vi "Field vs Slow IV v2.vi"() -> ()   [LabVIEW 2023]
uses:
  <vilib>/Utility/file.llb/Write Delimited Spreadsheet (DBL).vi
panel:
  in  "Tab Control 2":enum32{"cRIO", "Lockin", "Plot 2", "Plot 3"}(tab)
  out "I vs AI":cluster{"Y":dbl[], "Y":dbl[]}[](graph)=[{"Y"=[0.0, 0.01, 0.02, 0.03, 0.04, 0.05, 0.06, 0.07, 0.08, 0.09, 0.1, 0.11, 0.12, 0.13, 0.14, 0.15, 0.16, 0.17, 0.18, 0.19, 0.2, 0.21, 0.22, 0.23, 0.24, 0.25, 0.26, 0.27, 0.28, 0.29, 0.3, 0.31, 0.32, 0.33, 0.34, 0.35000000000000003, 0.36, 0.37, 0.38, 0.39, 0.4, 0.41000000000000003, 0.42, 0.43, 0.44, 0.45, 0.46, 0.47000000000000003, 0.48, 0.49, 0.5, 0.51, 0.52, 0.53, 0.54, 0.55, 0.56, 0.5700000000000001, 0.58, 0.59, 0.6, 0.61, 0.62, 0.63, 0.64, 0.65, 0.66, 0.67, 0.68, 0.6900000000000001, 0.7000000000000001, 0.71, 0.72, 0.73, 0.74, 0.75, 0.76, 0.77, 0.78, 0.79, 0.8, 0.81, 0.8200000000000001, 0.8300000000000001, 0.84, 0.85, 0.86, 0.87, 0.88, 0.89, 0.9, 0.91, 0.92, 0.93, 0.9400000000000001, 0.9500000000000001, 0.96, 0.97, 0.98, 0.99, 1.0, 1.01, 1.02, 1.03, 1.04, 1.05, 1.06, 1.07, 1.08, 1.09, 1.1, 1.11, 1.12, 1.1300000000000001, 1.1400000000000001, 1.1500000000000001, 1.16, 1.17, 1.18, 1.19, 1.2, 1.21, 1.22, 1.23, 1.24, 1.25, 1.26, 1.27, 1.28, 1.29, 1.3, 1.31, 1.32, 1.33, 1.34, 1.35, 1.36, 1.37, 1.3800000000000001, 1.3900000000000001, 1.4000000000000001, 1.41, 1.42, 1.43, 1.44, 1.45, 1.46, 1.47, 1.48, 1.49, 1.5, 1.51, 1.52, 1.53, 1.54, 1.55, 1.56, 1.57, 1.58, 1.59, 1.6, 1.61, 1.62, 1.6300000000000001, 1.6400000000000001, 1.6500000000000001, 1.6600000000000001, 1.67, 1.68, 1.69, 1.7, 1.71, 1.72, 1.73, 1.74, 1.75, 1.76, 1.77, 1.78, 1.79, 1.8, 1.81, 1.82, 1.83, 1.84, 1.85, 1.86, 1.87, 1.8800000000000001, 1.8900000000000001, 1.9000000000000001, 1.9100000000000001, 1.92, 1.93, 1.94, 1.95, 1.96, 1.97, 1.98, 1.99, 2.0, 2.0100000000000002, 2.02, 2.0300000000000002, 2.04, 2.05, 2.06, 2.07, 2.08, 2.09, 2.1, 2.11, 2.12, 2.13, 2.14, 2.15, 2.16, 2.17, 2.18, 2.19, 2.2, 2.21, 2.22, 2.23, 2.24, 2.25, 2.2600000000000002, 2.27, 2.2800000000000002, 2.29, 2.3000000000000003, 2.31, 2.32, 2.33, 2.34, 2.35, 2.36, 2.37, 2.38, 2.39, 2.4, 2.41, 2.42, 2.43, 2.44, 2.45, 2.46, 2.47, 2.48, 2.49, 2.5, 2.5100000000000002, 2.52, 2.5300000000000002, 2.54, 2.5500000000000003, 2.56, 2.57, 2.58, 2.59, 2.6, 2.61, 2.62, 2.63, 2.64, 2.65, 2.66, 2.67, 2.68, 2.69, 2.7, 2.71, 2.72, 2.73, 2.74, 2.75, 2.7600000000000002, 2.77, 2.7800000000000002, 2.79, 2.8000000000000003, 2.81, 2.82, 2.83, 2.84, 2.85, 2.86, 2.87, 2.88, 2.89, 2.9, 2.91, 2.92, 2.93, 2.94, 2.95, 2.96, 2.97, 2.98, 2.99, 3.0], "Y"=[2.09912109375e-05, 2.6015625e-05, 2.0756835937500003e-05, 2.4968261718750003e-05, 2.291015625e-05, 2.5644531250000002e-05, 2.3308105468750003e-05, 2.341796875e-05, 2.62646484375e-05, 2.48876953125e-05, 2.1000976562500003e-05, 2.4147949218750003e-05, 2.5754394531250003e-05, 2.3442382812500002e-05, 2.462890625e-05, 2.25537109375e-05, 2.5007324218750002e-05, 2.3037109375000003e-05, 2.2856445312500002e-05, 2.2717285156250002e-05, 2.41357421875e-05, 2.44873046875e-05, 2.4709472656250002e-05, 2.421630859375e-05, 2.6560058593750003e-05, 2.137451171875e-05, 2.361083984375e-05, 2.473876953125e-05, 1.990478515625e-05, 2.388427734375e-05, 2.21875e-05, 2.4270019531250003e-05, 2.480712890625e-05, 2.262451171875e-05, 2.370849609375e-05, 2.3144531250000002e-05, 2.422607421875e-05, 2.44775390625e-05, 2.233642578125e-05, 2.346923828125e-05, 2.3159179687500003e-05, 2.3681640625e-05, 2.5126953125000003e-05, 2.4238281250000002e-05, 2.0891113281250002e-05, 2.25927734375e-05, 2.1511230468750002e-05, 2.44482421875e-05, 2.1755371093750002e-05, 2.4130859375e-05, 2.342041015625e-05, 2.7426757812500002e-05, 2.2099609375e-05, 2.27001953125e-05, 2.5681152343750005e-05, 2.5070800781250004e-05, 2.67138671875e-05, 1.97119140625e-05, 2.027587890625e-05, 2.1047363281250002e-05, 2.325439453125e-05, 2.8649902343750002e-05, 2.2717285156250002e-05, 2.348876953125e-05, 2.63134765625e-05, 2.3552246093750003e-05, 2.6933593750000004e-05, 2.6767578125000004e-05, 2.558837890625e-05, 2.342041015625e-05, 2.642822265625e-05, 2.598388671875e-05, 2.4238281250000002e-05, 3.224609375e-05, 2.9941406250000003e-05, 3.089111328125e-05, 2.904541015625e-05, 4.072998046875e-05, 3.9006347656250006e-05, 4.6594238281250005e-05, 5.4602050781250004e-05, 5.186767578125e-05, 5.7617187500000004e-05, 5.64990234375e-05, 5.828125e-05, 6.0437011718750005e-05, 6.245361328125e-05, 6.554443359375e-05, 6.246826171875e-05, 6.654052734375e-05, 6.34423828125e-05, 6.683349609375e-05, 6.337158203124999e-05, 6.903076171875e-05, 7.051513671875001e-05, 6.797119140625e-05, 7.292724609375001e-05, 7.169433593750001e-05, 7.08251953125e-05, 7.458740234375e-05, 7.213134765625e-05, 7.000732421875e-05, 7.192626953125e-05, 7.560791015625e-05, 7.204833984375e-05, 7.61279296875e-05, 7.792236328125e-05, 7.745849609375e-05, 7.70068359375e-05, 7.795410156250001e-05, 8.091796875e-05, 8.347412109375e-05, 8.00830078125e-05, 7.839111328125001e-05, 8.351562500000001e-05, 8.119384765625e-05, 7.959716796875001e-05, 7.7822265625e-05, 8.2099609375e-05, 8.49853515625e-05, 8.425537109375001e-05, 8.463867187500001e-05, 8.37744140625e-05, 8.5576171875e-05, 8.346435546875e-05, 8.697509765625e-05, 8.865234375e-05, 8.927978515625e-05, 8.916748046875001e-05, 8.64404296875e-05, 9.275634765625001e-05, 9.026611328125001e-05, 9.218017578125e-05, 8.979003906250001e-05, 9.381103515625001e-05, 9.07177734375e-05, 9.376953125000001e-05, 9.364990234375001e-05, 9.407470703125001e-05, 9.20556640625e-05, 9.776611328125001e-05, 9.44970703125e-05, 9.7314453125e-05, 9.900390625e-05, 9.63671875e-05, 0.00010056884765625, 9.861572265625e-05, 0.00010073974609375001, 0.0001025146484375, 0.00010167480468750001, 0.0001015673828125, 0.00010302490234375, 0.00010155517578125, 0.00010652587890625001, 0.00010431152343750002, 0.0001023779296875, 0.0001060400390625, 0.00010368164062500001, 0.00010692382812500002, 0.0001058544921875, 0.0001072802734375, 0.00010769287109375001, 0.00010914306640625, 0.00010889892578125, 0.00010593505859375002, 0.00011151123046875001, 0.000111650390625, 0.00010907958984374999, 0.00011219482421875, 0.00010731201171875, 0.00011229248046875, 0.00011305664062500001, 0.0001139501953125, 0.00011421142578125001, 0.0001163134765625, 0.00011355224609375002, 0.000115390625, 0.0001179736328125, 0.000118828125, 0.00011745361328124999, 0.00012102294921875001, 0.00011634033203125002, 0.00011909912109375001, 0.00012057861328125, 0.00011787841796875001, 0.00012433349609375, 0.00012124267578125001, 0.00012028076171875, 0.00011879882812500001, 0.00012194335937500001, 0.0001228076171875, 0.00012369873046875, 0.00012751708984375, 0.00012575927734375002, 0.00012471923828125, 0.000126513671875, 0.0001298388671875, 0.00013156982421875003, 0.00013070068359375, 0.0001272998046875, 0.00013069091796875002, 0.00012986083984375003, 0.00013344970703125, 0.000129853515625, 0.00013442138671875, 0.00013176269531250002, 0.00013392822265625, 0.0001347265625, 0.0001333251953125, 0.00013612060546875, 0.0001330517578125, 0.00013523681640625, 0.00013681152343750002, 0.000135244140625, 0.00013745849609375, 0.00013937988281250002, 0.00013837646484375, 0.00014040771484375, 0.00014029785156250001, 0.00014124755859375, 0.00013885986328125, 0.00013990478515625001, 0.00013862060546875, 0.000142509765625, 0.00014126220703125002, 0.00014351318359375002, 0.00014447265625000002, 0.000145751953125, 0.00014315185546875, 0.00014501220703125, 0.00014614990234375, 0.0001438818359375, 0.00014447265625000002, 0.0001490283203125, 0.00014803466796875001, 0.0001479296875, 0.00014945800781250001, 0.0001504296875, 0.0001508837890625, 0.00015038085937500002, 0.00015168212890625, 0.00015281982421875, 0.00015464599609375, 0.0001536572265625, 0.00015431884765625, 0.00015674804687499999, 0.0001547314453125, 0.00015652587890625002, 0.00015684326171875001, 0.00015552734374999999, 0.00015493408203125003, 0.00015597900390625, 0.000159130859375, 0.00015770751953125, 0.00016166015625000002, 0.00016299560546875001, 0.00016100341796875, 0.00015983642578125, 0.00016435546875, 0.000161025390625, 0.0001635986328125, 0.0001652197265625, 0.00016124755859375, 0.00016710205078125, 0.00016457275390625, 0.00016589111328125, 0.000166328125, 0.0001637353515625, 0.00016878662109375, 0.00016859619140625, 0.0001676611328125, 0.00016881835937500002, 0.00016962646484375, 0.0001681005859375, 0.00017082031250000002, 0.00017445556640625, 0.0001698876953125, 0.0001721630859375, 0.00017332275390625001, 0.00017365966796875003, 0.0001742822265625, 0.000175556640625, 0.00017460937500000001, 0.00017539306640625003, 0.00017764404296875, 0.000178935546875, 0.00017882324218750003, 0.00018162353515625002, 0.00017995117187500002, 0.00017988037109375, 0.00017955566406250003, 0.00017959228515625002, 0.000180078125, 0.00018293212890625, 0.00017876953125, 0.00018194091796875001, 0.0001847021484375, 0.00018335205078125002, 0.000184111328125, 0.00018517822265625, 0.0001835205078125]}, ...(4 in all)]
  out "Name 0":string="DC Voltage V"
  out "I vs R":cluster{"Y":dbl[], "Y":dbl[]}[](graph)=[{"Y"=[0.0, 0.01, 0.02, 0.03, 0.04, 0.05, 0.06, 0.07, 0.08, 0.09, 0.1, 0.11, 0.12, 0.13, 0.14, 0.15, 0.16, 0.17, 0.18, 0.19, 0.2, 0.21, 0.22, 0.23, 0.24, 0.25, 0.26, 0.27, 0.28, 0.29, 0.3, 0.31, 0.32, 0.33, 0.34, 0.35000000000000003, 0.36, 0.37, 0.38, 0.39, 0.4, 0.41000000000000003, 0.42, 0.43, 0.44, 0.45, 0.46, 0.47000000000000003, 0.48, 0.49, 0.5, 0.51, 0.52, 0.53, 0.54, 0.55, 0.56, 0.5700000000000001, 0.58, 0.59, 0.6, 0.61, 0.62, 0.63, 0.64, 0.65, 0.66, 0.67, 0.68, 0.6900000000000001, 0.7000000000000001, 0.71, 0.72, 0.73, 0.74, 0.75, 0.76, 0.77, 0.78, 0.79, 0.8, 0.81, 0.8200000000000001, 0.8300000000000001, 0.84, 0.85, 0.86, 0.87, 0.88, 0.89, 0.9, 0.91, 0.92, 0.93, 0.9400000000000001, 0.9500000000000001, 0.96, 0.97, 0.98, 0.99, 1.0, 1.01, 1.02, 1.03, 1.04, 1.05, 1.06, 1.07, 1.08, 1.09, 1.1, 1.11, 1.12, 1.1300000000000001, 1.1400000000000001, 1.1500000000000001, 1.16, 1.17, 1.18, 1.19, 1.2, 1.21, 1.22, 1.23, 1.24, 1.25, 1.26, 1.27, 1.28, 1.29, 1.3, 1.31, 1.32, 1.33, 1.34, 1.35, 1.36, 1.37, 1.3800000000000001, 1.3900000000000001, 1.4000000000000001, 1.41, 1.42, 1.43, 1.44, 1.45, 1.46, 1.47, 1.48, 1.49, 1.5, 1.51, 1.52, 1.53, 1.54, 1.55, 1.56, 1.57, 1.58, 1.59, 1.6, 1.61, 1.62, 1.6300000000000001, 1.6400000000000001, 1.6500000000000001, 1.6600000000000001, 1.67, 1.68, 1.69, 1.7, 1.71, 1.72, 1.73, 1.74, 1.75, 1.76, 1.77, 1.78, 1.79, 1.8, 1.81, 1.82, 1.83, 1.84, 1.85, 1.86, 1.87, 1.8800000000000001, 1.8900000000000001, 1.9000000000000001, 1.9100000000000001, 1.92, 1.93, 1.94, 1.95, 1.96, 1.97, 1.98, 1.99, 2.0, 2.0100000000000002, 2.02, 2.0300000000000002, 2.04, 2.05, 2.06, 2.07, 2.08, 2.09, 2.1, 2.11, 2.12, 2.13, 2.14, 2.15, 2.16, 2.17, 2.18, 2.19, 2.2, 2.21, 2.22, 2.23, 2.24, 2.25, 2.2600000000000002, 2.27, 2.2800000000000002, 2.29, 2.3000000000000003, 2.31, 2.32, 2.33, 2.34, 2.35, 2.36, 2.37, 2.38, 2.39, 2.4, 2.41, 2.42, 2.43, 2.44, 2.45, 2.46, 2.47, 2.48, 2.49, 2.5, 2.5100000000000002, 2.52, 2.5300000000000002, 2.54, 2.5500000000000003, 2.56, 2.57, 2.58, 2.59, 2.6, 2.61, 2.62, 2.63, 2.64, 2.65, 2.66, 2.67, 2.68, 2.69, 2.7, 2.71, 2.72, 2.73, 2.74, 2.75, 2.7600000000000002, 2.77, 2.7800000000000002, 2.79, 2.8000000000000003, 2.81, 2.82, 2.83, 2.84, 2.85, 2.86, 2.87, 2.88, 2.89, 2.9, 2.91, 2.92, 2.93, 2.94, 2.95, 2.96, 2.97, 2.98, 2.99, 3.0], "Y"=[0.0, 0.0, 0.0, 0.0, 0.0, 0.0, 0.0, 0.0, 0.0, 0.0, 0.0, 0.0, 0.0, 0.0, 0.0, 0.0, 0.0, 0.0, 0.0, 0.0, 0.0, 0.0, 0.0, 0.0, 0.0, 0.0, 0.0, 0.0, 0.0, 0.0, 0.0, 0.0, 0.0, 0.0, 0.0, 0.0, 0.0, 0.0, 0.0, 0.0, 0.0, 0.0, 0.0, 0.0, 0.0, 0.0, 0.0, 0.0, 0.0, 0.0, 0.0, 0.0, 0.0, 0.0, 0.0, 0.0, 0.0, 0.0, 0.0, 0.0, 0.0, 0.0, 0.0, 0.0, 0.0, 0.0, 0.0, 0.0, 0.0, 0.0, 0.0, 0.0, 0.0, 0.0, 0.0, 0.0, 0.0, 0.0, 0.0, 0.0, 0.0, 0.0, 0.0, 0.0, 0.0, 0.0, 0.0, 0.0, 0.0, 0.0, 0.0, 0.0, 0.0, 0.0, 0.0, 0.0, 0.0, 0.0, 0.0, 0.0, 0.0, 0.0, 0.0, 0.0, 0.0, 0.0, 0.0, 0.0, 0.0, 0.0, 0.0, 0.0, 0.0, 0.0, 0.0, 0.0, 0.0, 0.0, 0.0, 0.0, 0.0, 0.0, 0.0, 0.0, 0.0, 0.0, 0.0, 0.0, 0.0, 0.0, 0.0, 0.0, 0.0, 0.0, 0.0, 0.0, 0.0, 0.0, 0.0, 0.0, 0.0, 0.0, 0.0, 0.0, 0.0, 0.0, 0.0, 0.0, 0.0, 0.0, 0.0, 0.0, 0.0, 0.0, 0.0, 0.0, 0.0, 0.0, 0.0, 0.0, 0.0, 0.0, 0.0, 0.0, 0.0, 0.0, 0.0, 0.0, 0.0, 0.0, 0.0, 0.0, 0.0, 0.0, 0.0, 0.0, 0.0, 0.0, 0.0, 0.0, 0.0, 0.0, 0.0, 0.0, 0.0, 0.0, 0.0, 0.0, 0.0, 0.0, 0.0, 0.0, 0.0, 0.0, 0.0, 0.0, 0.0, 0.0, 0.0, 0.0, 0.0, 0.0, 0.0, 0.0, 0.0, 0.0, 0.0, 0.0, 0.0, 0.0, 0.0, 0.0, 0.0, 0.0, 0.0, 0.0, 0.0, 0.0, 0.0, 0.0, 0.0, 0.0, 0.0, 0.0, 0.0, 0.0, 0.0, 0.0, 0.0, 0.0, 0.0, 0.0, 0.0, 0.0, 0.0, 0.0, 0.0, 0.0, 0.0, 0.0, 0.0, 0.0, 0.0, 0.0, 0.0, 0.0, 0.0, 0.0, 0.0, 0.0, 0.0, 0.0, 0.0, 0.0, 0.0, 0.0, 0.0, 0.0, 0.0, 0.0, 0.0, 0.0, 0.0, 0.0, 0.0, 0.0, 0.0, 0.0, 0.0, 0.0, 0.0, 0.0, 0.0, 0.0, 0.0, 0.0, 0.0, 0.0, 0.0, 0.0, 0.0, 0.0, 0.0, 0.0, 0.0, 0.0, 0.0, 0.0, 0.0, 0.0, 0.0, 0.0, 0.0, 0.0, 0.0, 0.0, 0.0, 0.0, 0.0, 0.0, 0.0]}, {"Y"=[0.0, 0.01, 0.02, 0.03, 0.04, 0.05, 0.06, 0.07, 0.08, 0.09, 0.1, 0.11, 0.12, 0.13, 0.14, 0.15, 0.16, 0.17, 0.18, 0.19, 0.2, 0.21, 0.22, 0.23, 0.24, 0.25, 0.26, 0.27, 0.28, 0.29, 0.3, 0.31, 0.32, 0.33, 0.34, 0.35000000000000003, 0.36, 0.37, 0.38, 0.39, 0.4, 0.41000000000000003, 0.42, 0.43, 0.44, 0.45, 0.46, 0.47000000000000003, 0.48, 0.49, 0.5, 0.51, 0.52, 0.53, 0.54, 0.55, 0.56, 0.5700000000000001, 0.58, 0.59, 0.6, 0.61, 0.62, 0.63, 0.64, 0.65, 0.66, 0.67, 0.68, 0.6900000000000001, 0.7000000000000001, 0.71, 0.72, 0.73, 0.74, 0.75, 0.76, 0.77, 0.78, 0.79, 0.8, 0.81, 0.8200000000000001, 0.8300000000000001, 0.84, 0.85, 0.86, 0.87, 0.88, 0.89, 0.9, 0.91, 0.92, 0.93, 0.9400000000000001, 0.9500000000000001, 0.96, 0.97, 0.98, 0.99, 1.0, 1.01, 1.02, 1.03, 1.04, 1.05, 1.06, 1.07, 1.08, 1.09, 1.1, 1.11, 1.12, 1.1300000000000001, 1.1400000000000001, 1.1500000000000001, 1.16, 1.17, 1.18, 1.19, 1.2, 1.21, 1.22, 1.23, 1.24, 1.25, 1.26, 1.27, 1.28, 1.29, 1.3, 1.31, 1.32, 1.33, 1.34, 1.35, 1.36, 1.37, 1.3800000000000001, 1.3900000000000001, 1.4000000000000001, 1.41, 1.42, 1.43, 1.44, 1.45, 1.46, 1.47, 1.48, 1.49, 1.5, 1.51, 1.52, 1.53, 1.54, 1.55, 1.56, 1.57, 1.58, 1.59, 1.6, 1.61, 1.62, 1.6300000000000001, 1.6400000000000001, 1.6500000000000001, 1.6600000000000001, 1.67, 1.68, 1.69, 1.7, 1.71, 1.72, 1.73, 1.74, 1.75, 1.76, 1.77, 1.78, 1.79, 1.8, 1.81, 1.82, 1.83, 1.84, 1.85, 1.86, 1.87, 1.8800000000000001, 1.8900000000000001, 1.9000000000000001, 1.9100000000000001, 1.92, 1.93, 1.94, 1.95, 1.96, 1.97, 1.98, 1.99, 2.0, 2.0100000000000002, 2.02, 2.0300000000000002, 2.04, 2.05, 2.06, 2.07, 2.08, 2.09, 2.1, 2.11, 2.12, 2.13, 2.14, 2.15, 2.16, 2.17, 2.18, 2.19, 2.2, 2.21, 2.22, 2.23, 2.24, 2.25, 2.2600000000000002, 2.27, 2.2800000000000002, 2.29, 2.3000000000000003, 2.31, 2.32, 2.33, 2.34, 2.35, 2.36, 2.37, 2.38, 2.39, 2.4, 2.41, 2.42, 2.43, 2.44, 2.45, 2.46, 2.47, 2.48, 2.49, 2.5, 2.5100000000000002, 2.52, 2.5300000000000002, 2.54, 2.5500000000000003, 2.56, 2.57, 2.58, 2.59, 2.6, 2.61, 2.62, 2.63, 2.64, 2.65, 2.66, 2.67, 2.68, 2.69, 2.7, 2.71, 2.72, 2.73, 2.74, 2.75, 2.7600000000000002, 2.77, 2.7800000000000002, 2.79, 2.8000000000000003, 2.81, 2.82, 2.83, 2.84, 2.85, 2.86, 2.87, 2.88, 2.89, 2.9, 2.91, 2.92, 2.93, 2.94, 2.95, 2.96, 2.97, 2.98, 2.99, 3.0], "Y"=[0.0, 0.0, 0.0, 0.0, 0.0, 0.0, 0.0, 0.0, 0.0, 0.0, 0.0, 0.0, 0.0, 0.0, 0.0, 0.0, 0.0, 0.0, 0.0, 0.0, 0.0, 0.0, 0.0, 0.0, 0.0, 0.0, 0.0, 0.0, 0.0, 0.0, 0.0, 0.0, 0.0, 0.0, 0.0, 0.0, 0.0, 0.0, 0.0, 0.0, 0.0, 0.0, 0.0, 0.0, 0.0, 0.0, 0.0, 0.0, 0.0, 0.0, 0.0, 0.0, 0.0, 0.0, 0.0, 0.0, 0.0, 0.0, 0.0, 0.0, 0.0, 0.0, 0.0, 0.0, 0.0, 0.0, 0.0, 0.0, 0.0, 0.0, 0.0, 0.0, 0.0, 0.0, 0.0, 0.0, 0.0, 0.0, 0.0, 0.0, 0.0, 0.0, 0.0, 0.0, 0.0, 0.0, 0.0, 0.0, 0.0, 0.0, 0.0, 0.0, 0.0, 0.0, 0.0, 0.0, 0.0, 0.0, 0.0, 0.0, 0.0, 0.0, 0.0, 0.0, 0.0, 0.0, 0.0, 0.0, 0.0, 0.0, 0.0, 0.0, 0.0, 0.0, 0.0, 0.0, 0.0, 0.0, 0.0, 0.0, 0.0, 0.0, 0.0, 0.0, 0.0, 0.0, 0.0, 0.0, 0.0, 0.0, 0.0, 0.0, 0.0, 0.0, 0.0, 0.0, 0.0, 0.0, 0.0, 0.0, 0.0, 0.0, 0.0, 0.0, 0.0, 0.0, 0.0, 0.0, 0.0, 0.0, 0.0, 0.0, 0.0, 0.0, 0.0, 0.0, 0.0, 0.0, 0.0, 0.0, 0.0, 0.0, 0.0, 0.0, 0.0, 0.0, 0.0, 0.0, 0.0, 0.0, 0.0, 0.0, 0.0, 0.0, 0.0, 0.0, 0.0, 0.0, 0.0, 0.0, 0.0, 0.0, 0.0, 0.0, 0.0, 0.0, 0.0, 0.0, 0.0, 0.0, 0.0, 0.0, 0.0, 0.0, 0.0, 0.0, 0.0, 0.0, 0.0, 0.0, 0.0, 0.0, 0.0, 0.0, 0.0, 0.0, 0.0, 0.0, 0.0, 0.0, 0.0, 0.0, 0.0, 0.0, 0.0, 0.0, 0.0, 0.0, 0.0, 0.0, 0.0, 0.0, 0.0, 0.0, 0.0, 0.0, 0.0, 0.0, 0.0, 0.0, 0.0, 0.0, 0.0, 0.0, 0.0, 0.0, 0.0, 0.0, 0.0, 0.0, 0.0, 0.0, 0.0, 0.0, 0.0, 0.0, 0.0, 0.0, 0.0, 0.0, 0.0, 0.0, 0.0, 0.0, 0.0, 0.0, 0.0, 0.0, 0.0, 0.0, 0.0, 0.0, 0.0, 0.0, 0.0, 0.0, 0.0, 0.0, 0.0, 0.0, 0.0, 0.0, 0.0, 0.0, 0.0, 0.0, 0.0, 0.0, 0.0, 0.0, 0.0, 0.0, 0.0, 0.0, 0.0, 0.0, 0.0, 0.0, 0.0, 0.0, 0.0, 0.0, 0.0, 0.0, 0.0, 0.0, 0.0, 0.0, 0.0, 0.0, 0.0]}, {"Y"=[0.0, 0.01, 0.02, 0.03, 0.04, 0.05, 0.06, 0.07, 0.08, 0.09, 0.1, 0.11, 0.12, 0.13, 0.14, 0.15, 0.16, 0.17, 0.18, 0.19, 0.2, 0.21, 0.22, 0.23, 0.24, 0.25, 0.26, 0.27, 0.28, 0.29, 0.3, 0.31, 0.32, 0.33, 0.34, 0.35000000000000003, 0.36, 0.37, 0.38, 0.39, 0.4, 0.41000000000000003, 0.42, 0.43, 0.44, 0.45, 0.46, 0.47000000000000003, 0.48, 0.49, 0.5, 0.51, 0.52, 0.53, 0.54, 0.55, 0.56, 0.5700000000000001, 0.58, 0.59, 0.6, 0.61, 0.62, 0.63, 0.64, 0.65, 0.66, 0.67, 0.68, 0.6900000000000001, 0.7000000000000001, 0.71, 0.72, 0.73, 0.74, 0.75, 0.76, 0.77, 0.78, 0.79, 0.8, 0.81, 0.8200000000000001, 0.8300000000000001, 0.84, 0.85, 0.86, 0.87, 0.88, 0.89, 0.9, 0.91, 0.92, 0.93, 0.9400000000000001, 0.9500000000000001, 0.96, 0.97, 0.98, 0.99, 1.0, 1.01, 1.02, 1.03, 1.04, 1.05, 1.06, 1.07, 1.08, 1.09, 1.1, 1.11, 1.12, 1.1300000000000001, 1.1400000000000001, 1.1500000000000001, 1.16, 1.17, 1.18, 1.19, 1.2, 1.21, 1.22, 1.23, 1.24, 1.25, 1.26, 1.27, 1.28, 1.29, 1.3, 1.31, 1.32, 1.33, 1.34, 1.35, 1.36, 1.37, 1.3800000000000001, 1.3900000000000001, 1.4000000000000001, 1.41, 1.42, 1.43, 1.44, 1.45, 1.46, 1.47, 1.48, 1.49, 1.5, 1.51, 1.52, 1.53, 1.54, 1.55, 1.56, 1.57, 1.58, 1.59, 1.6, 1.61, 1.62, 1.6300000000000001, 1.6400000000000001, 1.6500000000000001, 1.6600000000000001, 1.67, 1.68, 1.69, 1.7, 1.71, 1.72, 1.73, 1.74, 1.75, 1.76, 1.77, 1.78, 1.79, 1.8, 1.81, 1.82, 1.83, 1.84, 1.85, 1.86, 1.87, 1.8800000000000001, 1.8900000000000001, 1.9000000000000001, 1.9100000000000001, 1.92, 1.93, 1.94, 1.95, 1.96, 1.97, 1.98, 1.99, 2.0, 2.0100000000000002, 2.02, 2.0300000000000002, 2.04, 2.05, 2.06, 2.07, 2.08, 2.09, 2.1, 2.11, 2.12, 2.13, 2.14, 2.15, 2.16, 2.17, 2.18, 2.19, 2.2, 2.21, 2.22, 2.23, 2.24, 2.25, 2.2600000000000002, 2.27, 2.2800000000000002, 2.29, 2.3000000000000003, 2.31, 2.32, 2.33, 2.34, 2.35, 2.36, 2.37, 2.38, 2.39, 2.4, 2.41, 2.42, 2.43, 2.44, 2.45, 2.46, 2.47, 2.48, 2.49, 2.5, 2.5100000000000002, 2.52, 2.5300000000000002, 2.54, 2.5500000000000003, 2.56, 2.57, 2.58, 2.59, 2.6, 2.61, 2.62, 2.63, 2.64, 2.65, 2.66, 2.67, 2.68, 2.69, 2.7, 2.71, 2.72, 2.73, 2.74, 2.75, 2.7600000000000002, 2.77, 2.7800000000000002, 2.79, 2.8000000000000003, 2.81, 2.82, 2.83, 2.84, 2.85, 2.86, 2.87, 2.88, 2.89, 2.9, 2.91, 2.92, 2.93, 2.94, 2.95, 2.96, 2.97, 2.98, 2.99, 3.0], "Y"=[0.0, 0.0, 0.0, 0.0, 0.0, 0.0, 0.0, 0.0, 0.0, 0.0, 0.0, 0.0, 0.0, 0.0, 0.0, 0.0, 0.0, 0.0, 0.0, 0.0, 0.0, 0.0, 0.0, 0.0, 0.0, 0.0, 0.0, 0.0, 0.0, 0.0, 0.0, 0.0, 0.0, 0.0, 0.0, 0.0, 0.0, 0.0, 0.0, 0.0, 0.0, 0.0, 0.0, 0.0, 0.0, 0.0, 0.0, 0.0, 0.0, 0.0, 0.0, 0.0, 0.0, 0.0, 0.0, 0.0, 0.0, 0.0, 0.0, 0.0, 0.0, 0.0, 0.0, 0.0, 0.0, 0.0, 0.0, 0.0, 0.0, 0.0, 0.0, 0.0, 0.0, 0.0, 0.0, 0.0, 0.0, 0.0, 0.0, 0.0, 0.0, 0.0, 0.0, 0.0, 0.0, 0.0, 0.0, 0.0, 0.0, 0.0, 0.0, 0.0, 0.0, 0.0, 0.0, 0.0, 0.0, 0.0, 0.0, 0.0, 0.0, 0.0, 0.0, 0.0, 0.0, 0.0, 0.0, 0.0, 0.0, 0.0, 0.0, 0.0, 0.0, 0.0, 0.0, 0.0, 0.0, 0.0, 0.0, 0.0, 0.0, 0.0, 0.0, 0.0, 0.0, 0.0, 0.0, 0.0, 0.0, 0.0, 0.0, 0.0, 0.0, 0.0, 0.0, 0.0, 0.0, 0.0, 0.0, 0.0, 0.0, 0.0, 0.0, 0.0, 0.0, 0.0, 0.0, 0.0, 0.0, 0.0, 0.0, 0.0, 0.0, 0.0, 0.0, 0.0, 0.0, 0.0, 0.0, 0.0, 0.0, 0.0, 0.0, 0.0, 0.0, 0.0, 0.0, 0.0, 0.0, 0.0, 0.0, 0.0, 0.0, 0.0, 0.0, 0.0, 0.0, 0.0, 0.0, 0.0, 0.0, 0.0, 0.0, 0.0, 0.0, 0.0, 0.0, 0.0, 0.0, 0.0, 0.0, 0.0, 0.0, 0.0, 0.0, 0.0, 0.0, 0.0, 0.0, 0.0, 0.0, 0.0, 0.0, 0.0, 0.0, 0.0, 0.0, 0.0, 0.0, 0.0, 0.0, 0.0, 0.0, 0.0, 0.0, 0.0, 0.0, 0.0, 0.0, 0.0, 0.0, 0.0, 0.0, 0.0, 0.0, 0.0, 0.0, 0.0, 0.0, 0.0, 0.0, 0.0, 0.0, 0.0, 0.0, 0.0, 0.0, 0.0, 0.0, 0.0, 0.0, 0.0, 0.0, 0.0, 0.0, 0.0, 0.0, 0.0, 0.0, 0.0, 0.0, 0.0, 0.0, 0.0, 0.0, 0.0, 0.0, 0.0, 0.0, 0.0, 0.0, 0.0, 0.0, 0.0, 0.0, 0.0, 0.0, 0.0, 0.0, 0.0, 0.0, 0.0, 0.0, 0.0, 0.0, 0.0, 0.0, 0.0, 0.0, 0.0, 0.0, 0.0, 0.0, 0.0, 0.0, 0.0, 0.0, 0.0, 0.0, 0.0, 0.0, 0.0, 0.0, 0.0, 0.0, 0.0, 0.0, 0.0, 0.0, 0.0, 0.0]}, {"Y"=[0.0, 0.01, 0.02, 0.03, 0.04, 0.05, 0.06, 0.07, 0.08, 0.09, 0.1, 0.11, 0.12, 0.13, 0.14, 0.15, 0.16, 0.17, 0.18, 0.19, 0.2, 0.21, 0.22, 0.23, 0.24, 0.25, 0.26, 0.27, 0.28, 0.29, 0.3, 0.31, 0.32, 0.33, 0.34, 0.35000000000000003, 0.36, 0.37, 0.38, 0.39, 0.4, 0.41000000000000003, 0.42, 0.43, 0.44, 0.45, 0.46, 0.47000000000000003, 0.48, 0.49, 0.5, 0.51, 0.52, 0.53, 0.54, 0.55, 0.56, 0.5700000000000001, 0.58, 0.59, 0.6, 0.61, 0.62, 0.63, 0.64, 0.65, 0.66, 0.67, 0.68, 0.6900000000000001, 0.7000000000000001, 0.71, 0.72, 0.73, 0.74, 0.75, 0.76, 0.77, 0.78, 0.79, 0.8, 0.81, 0.8200000000000001, 0.8300000000000001, 0.84, 0.85, 0.86, 0.87, 0.88, 0.89, 0.9, 0.91, 0.92, 0.93, 0.9400000000000001, 0.9500000000000001, 0.96, 0.97, 0.98, 0.99, 1.0, 1.01, 1.02, 1.03, 1.04, 1.05, 1.06, 1.07, 1.08, 1.09, 1.1, 1.11, 1.12, 1.1300000000000001, 1.1400000000000001, 1.1500000000000001, 1.16, 1.17, 1.18, 1.19, 1.2, 1.21, 1.22, 1.23, 1.24, 1.25, 1.26, 1.27, 1.28, 1.29, 1.3, 1.31, 1.32, 1.33, 1.34, 1.35, 1.36, 1.37, 1.3800000000000001, 1.3900000000000001, 1.4000000000000001, 1.41, 1.42, 1.43, 1.44, 1.45, 1.46, 1.47, 1.48, 1.49, 1.5, 1.51, 1.52, 1.53, 1.54, 1.55, 1.56, 1.57, 1.58, 1.59, 1.6, 1.61, 1.62, 1.6300000000000001, 1.6400000000000001, 1.6500000000000001, 1.6600000000000001, 1.67, 1.68, 1.69, 1.7, 1.71, 1.72, 1.73, 1.74, 1.75, 1.76, 1.77, 1.78, 1.79, 1.8, 1.81, 1.82, 1.83, 1.84, 1.85, 1.86, 1.87, 1.8800000000000001, 1.8900000000000001, 1.9000000000000001, 1.9100000000000001, 1.92, 1.93, 1.94, 1.95, 1.96, 1.97, 1.98, 1.99, 2.0, 2.0100000000000002, 2.02, 2.0300000000000002, 2.04, 2.05, 2.06, 2.07, 2.08, 2.09, 2.1, 2.11, 2.12, 2.13, 2.14, 2.15, 2.16, 2.17, 2.18, 2.19, 2.2, 2.21, 2.22, 2.23, 2.24, 2.25, 2.2600000000000002, 2.27, 2.2800000000000002, 2.29, 2.3000000000000003, 2.31, 2.32, 2.33, 2.34, 2.35, 2.36, 2.37, 2.38, 2.39, 2.4, 2.41, 2.42, 2.43, 2.44, 2.45, 2.46, 2.47, 2.48, 2.49, 2.5, 2.5100000000000002, 2.52, 2.5300000000000002, 2.54, 2.5500000000000003, 2.56, 2.57, 2.58, 2.59, 2.6, 2.61, 2.62, 2.63, 2.64, 2.65, 2.66, 2.67, 2.68, 2.69, 2.7, 2.71, 2.72, 2.73, 2.74, 2.75, 2.7600000000000002, 2.77, 2.7800000000000002, 2.79, 2.8000000000000003, 2.81, 2.82, 2.83, 2.84, 2.85, 2.86, 2.87, 2.88, 2.89, 2.9, 2.91, 2.92, 2.93, 2.94, 2.95, 2.96, 2.97, 2.98, 2.99, 3.0], "Y"=[0.0, 0.0, 0.0, 0.0, 0.0, 0.0, 0.0, 0.0, 0.0, 0.0, 0.0, 0.0, 0.0, 0.0, 0.0, 0.0, 0.0, 0.0, 0.0, 0.0, 0.0, 0.0, 0.0, 0.0, 0.0, 0.0, 0.0, 0.0, 0.0, 0.0, 0.0, 0.0, 0.0, 0.0, 0.0, 0.0, 0.0, 0.0, 0.0, 0.0, 0.0, 0.0, 0.0, 0.0, 0.0, 0.0, 0.0, 0.0, 0.0, 0.0, 0.0, 0.0, 0.0, 0.0, 0.0, 0.0, 0.0, 0.0, 0.0, 0.0, 0.0, 0.0, 0.0, 0.0, 0.0, 0.0, 0.0, 0.0, 0.0, 0.0, 0.0, 0.0, 0.0, 0.0, 0.0, 0.0, 0.0, 0.0, 0.0, 0.0, 0.0, 0.0, 0.0, 0.0, 0.0, 0.0, 0.0, 0.0, 0.0, 0.0, 0.0, 0.0, 0.0, 0.0, 0.0, 0.0, 0.0, 0.0, 0.0, 0.0, 0.0, 0.0, 0.0, 0.0, 0.0, 0.0, 0.0, 0.0, 0.0, 0.0, 0.0, 0.0, 0.0, 0.0, 0.0, 0.0, 0.0, 0.0, 0.0, 0.0, 0.0, 0.0, 0.0, 0.0, 0.0, 0.0, 0.0, 0.0, 0.0, 0.0, 0.0, 0.0, 0.0, 0.0, 0.0, 0.0, 0.0, 0.0, 0.0, 0.0, 0.0, 0.0, 0.0, 0.0, 0.0, 0.0, 0.0, 0.0, 0.0, 0.0, 0.0, 0.0, 0.0, 0.0, 0.0, 0.0, 0.0, 0.0, 0.0, 0.0, 0.0, 0.0, 0.0, 0.0, 0.0, 0.0, 0.0, 0.0, 0.0, 0.0, 0.0, 0.0, 0.0, 0.0, 0.0, 0.0, 0.0, 0.0, 0.0, 0.0, 0.0, 0.0, 0.0, 0.0, 0.0, 0.0, 0.0, 0.0, 0.0, 0.0, 0.0, 0.0, 0.0, 0.0, 0.0, 0.0, 0.0, 0.0, 0.0, 0.0, 0.0, 0.0, 0.0, 0.0, 0.0, 0.0, 0.0, 0.0, 0.0, 0.0, 0.0, 0.0, 0.0, 0.0, 0.0, 0.0, 0.0, 0.0, 0.0, 0.0, 0.0, 0.0, 0.0, 0.0, 0.0, 0.0, 0.0, 0.0, 0.0, 0.0, 0.0, 0.0, 0.0, 0.0, 0.0, 0.0, 0.0, 0.0, 0.0, 0.0, 0.0, 0.0, 0.0, 0.0, 0.0, 0.0, 0.0, 0.0, 0.0, 0.0, 0.0, 0.0, 0.0, 0.0, 0.0, 0.0, 0.0, 0.0, 0.0, 0.0, 0.0, 0.0, 0.0, 0.0, 0.0, 0.0, 0.0, 0.0, 0.0, 0.0, 0.0, 0.0, 0.0, 0.0, 0.0, 0.0, 0.0, 0.0, 0.0, 0.0, 0.0, 0.0, 0.0, 0.0, 0.0, 0.0, 0.0, 0.0, 0.0, 0.0, 0.0, 0.0, 0.0, 0.0, 0.0, 0.0, 0.0, 0.0, 0.0, 0.0, 0.0]}]
  out "Name 1":string="DC current uA"
  out "Name 2":string="dV V"
  out "Name 3":string="dI uA"
  in  "Tab Control":T1(tab)=enum."Data log and Status"
  in  "cRIO IP":string="//172.22.11.2"
  in  "Reading Average times":i32=10
  in  "Current Start uA":dbl
  in  "Current Range uA":dbl=3.0
  in  "Current Step uA":dbl=0.01
  in  "Current output Scale factor":dbl=1.0
  in  "Ramp type":string(combo)="Range"
  in  "Ramp up first T":bool=TRUE
  in  "AO Channel":string(combo)="AO0"
  in  "Delay Time s":dbl=0.1 caption="Delay Time (s)"
  in  "Channel name 0":string(combo)="DC Voltage V"
  in  "Scale factor0":dbl=0.0001
  in  "Chan 1":bool=TRUE
  in  "Channel name 1":string(combo)="DC current uA"
  in  "Scale factor1":dbl=1.0
  in  "Chan 2":bool
  in  "Channel name 2":string(combo)="dV V"
  in  "Scale factor2":dbl=1.0
  in  "Chan 3":bool
  in  "Channel name 3":string(combo)="dI uA"
  in  "Scale factor3":dbl=1.0
  in  "Lockin Chan name 1":string(combo)="Voltage mV"
  in  "Lockin Chan name 2":string(combo)="Current mV"
  in  "Use Lockin":bool
  in  "Lockin 1":bool
  in  "Lockin 2":bool
  in  "Lockin address 1":string="GPIB0::8::INSTR"
  in  "Lockin address 2":string="GPIB0::9::INSTR"
  in  "Lockin Status":string
  in  "Contour plot folder":path=path "C:/Users/gyue/Desktop/20221209 G22L measurement"
  in  "Book name":string="book786"
  in  "Current VI path":path=path "C:/Users/gyue/Desktop/General-Measurement/cRIO related/Field vs Slow IV v2.vi"
  out "Current Field mT":dbl=0.6000000000000001
  in  "stop":bool
  out "error out":errorcluster
  in  "Ramp up first T 2":bool=TRUE
  in  "Ramp type 2":string(combo)="Range"
  in  "Field Origin mT":dbl=-1.0 format="%#_13g"
  in  "Field step mT":dbl=0.1 format="%#_13g"
  in  "Field Radius mT":dbl=1.6 format="%#_13g"
  in  "Field Rate mT per sec":dbl=0.1 format="%#_13g"
  in  "Magnet Device Select":string(combo)="Elsa Magnet mT"
  # "Voltage x factor=uA"
  # "Voltage x factor=actual"
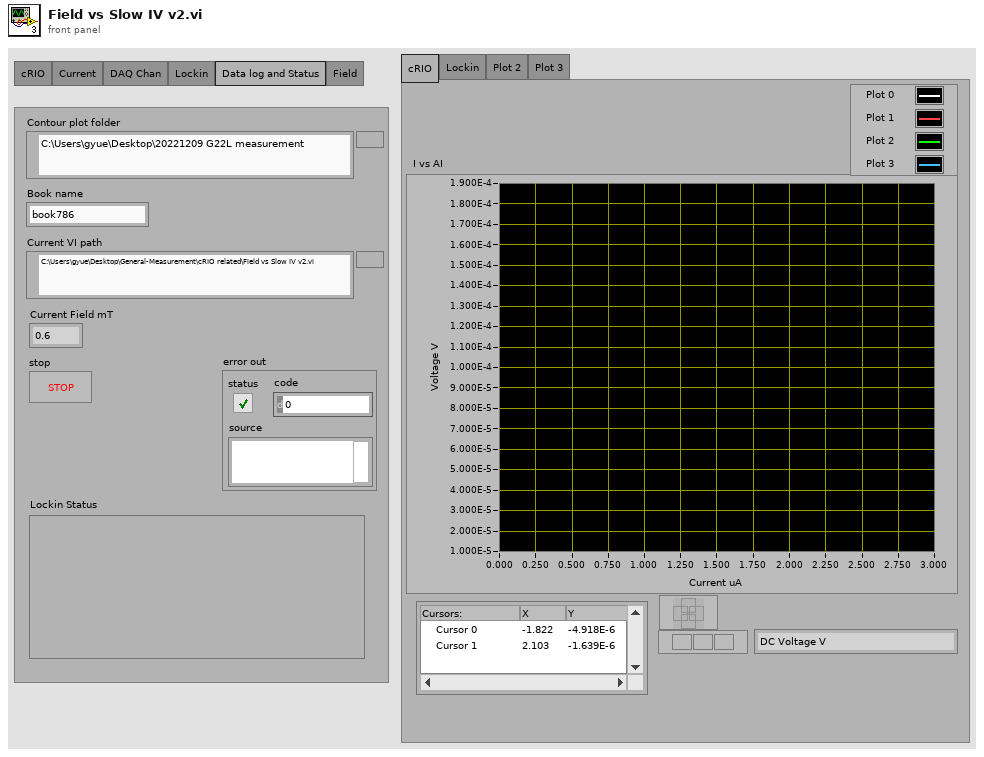
[diagram p1: front panel]
types:
  T1 = enum32{"cRIO", "Current", "DAQ Chan", "Lockin", "Data log and Status", "Field"}
  T2 = cluster{"AI0":dbl, "AI1":dbl, "AI2":dbl, "AI3":dbl}
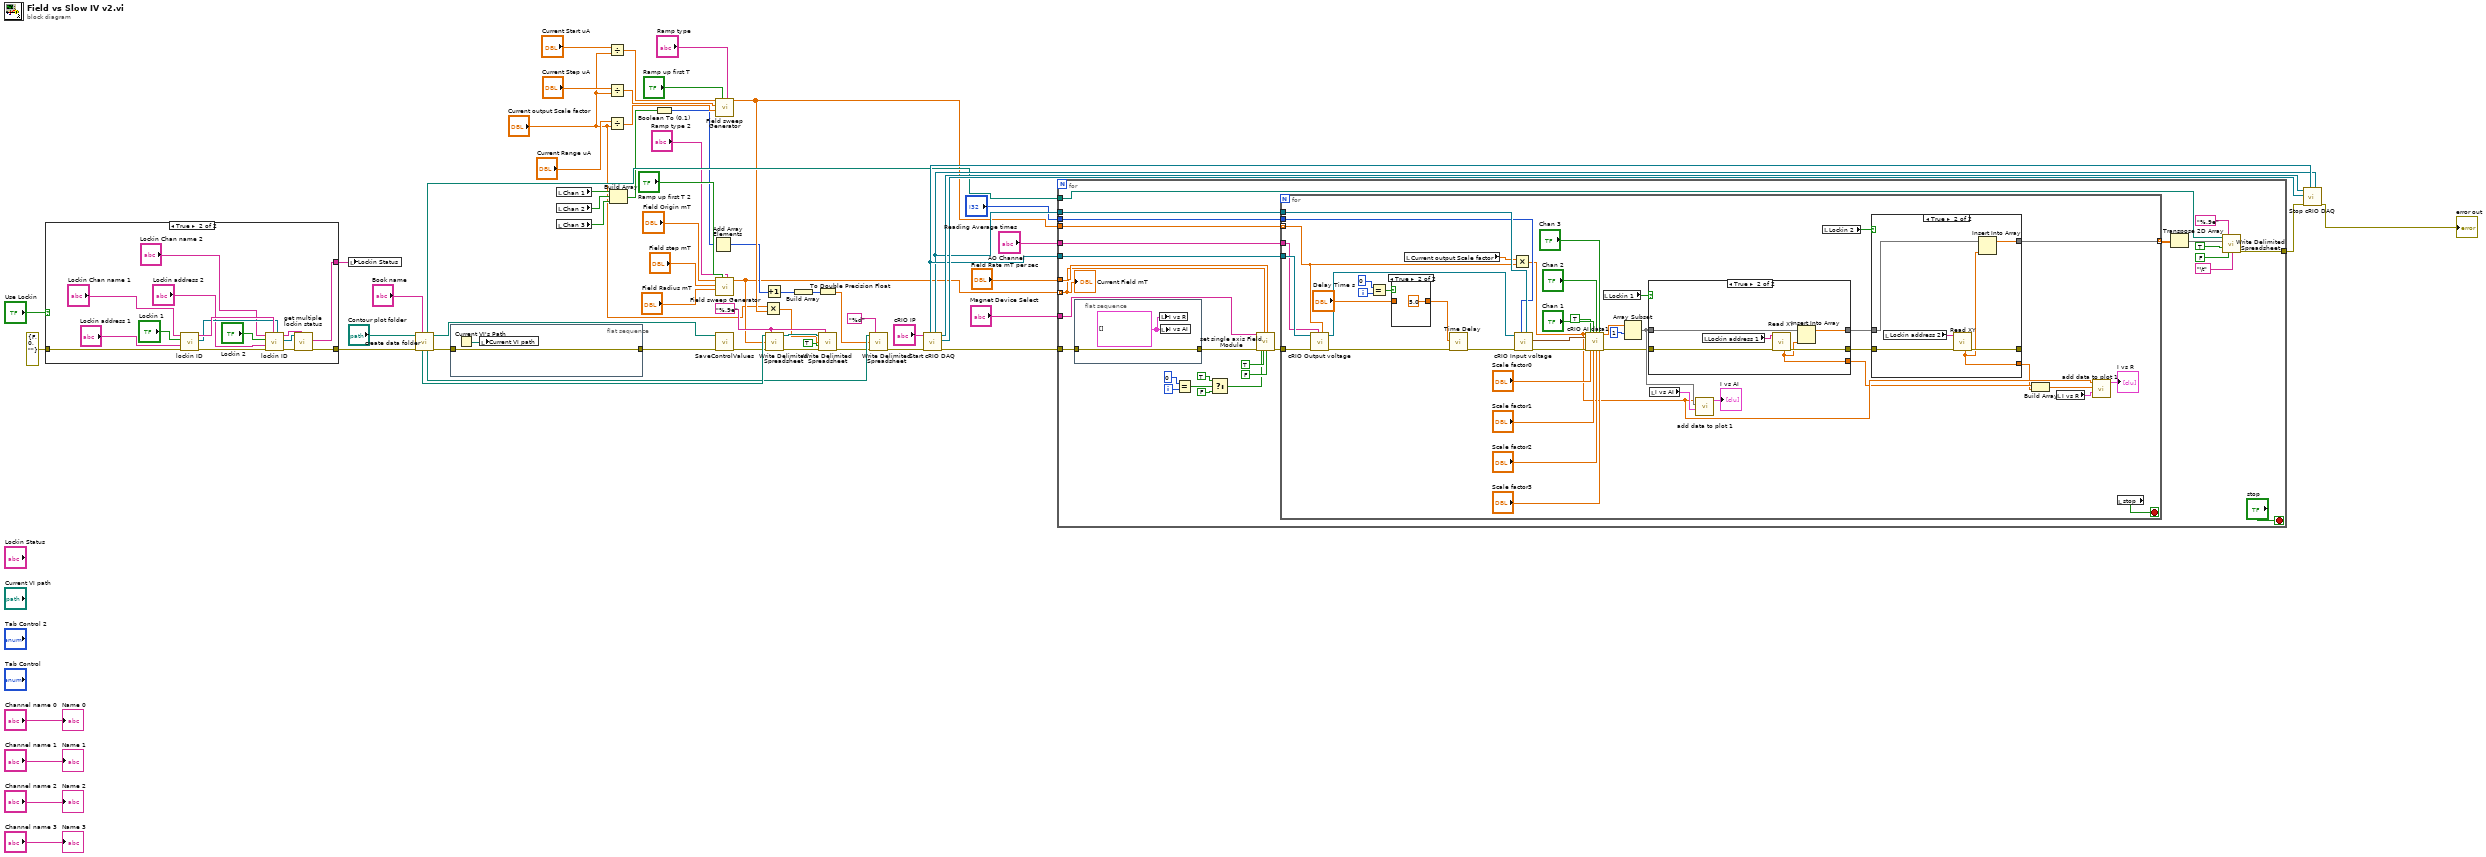
[diagram p0: block diagram]
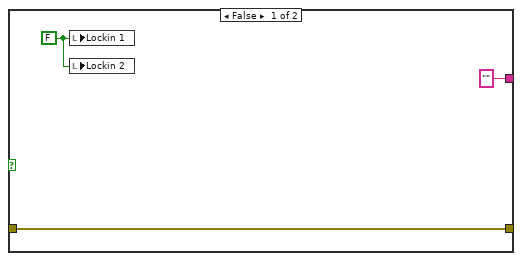
[diagram p2: hidden frame]
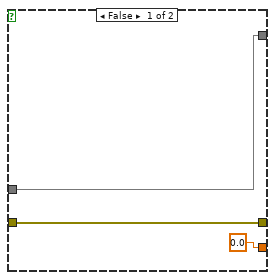
[diagram p3: hidden frame]
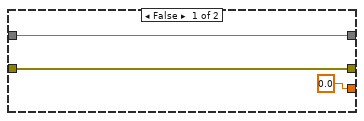
[diagram p4: hidden frame]
diagram:
  w28 = "%.9e" ("format (%.3f)")
  n1 = case shown="True" "Use Lockin" {
    tunnel: ["" ("Status output") w66] -> w3
    tunnel: [w65 w80] -> w2
    tunnel: errorcluster {"status"=FALSE, "code"=0, "source"=""} ("error in") -> [w65 w79]
    frame False {
      w63 = FALSE ("Lockin 1")
      n2 = local write "Lockin 1"(w63) -> ()
      n3 = local write "Lockin 2"(w63) -> ()
    }
    frame True {
      n4 = call "lockin ID.vi"("error in (no error)"=w79, "Lockin address"="Lockin address 1", "Lockin on"="Lockin 1", "Lockin Chan name"="Lockin Chan name 1") -> ("error out"=w78:errorcluster, "Addresses out"=w73:refnum<visa-resource-name>[], "names out"=w74:string[])  [unwired: 5 in]
      n5 = call "lockin ID.vi"("Addresses IN"=w73, "names in"=w74, "error in (no error)"=w78, "Lockin address"="Lockin address 2", "Lockin on"="Lockin 2", "Lockin Chan name"="Lockin Chan name 2") -> ("error out"=w67:errorcluster, "Addresses out"=w68:refnum<visa-resource-name>[], "names out"=w69:string[])  [unwired: 3 in]
      n6 = call "get multiple lockin status.vi"("Device channel names"=w69, "error in (no error)"=w67, "SRS830 addresses"=w68) -> ("error out"=w80:errorcluster, "Status output"=w66:string)  [unwired: 6 in, 1 out]
    }
  }
  n7 = local write "Lockin Status"(w3) -> ()
  n8 = call "create data folder.vi"("Book name"="Book name", "error in"=w2, "Contour plot folder"="Contour plot folder") -> ("error out"=w37:errorcluster, "xml path"=w39:path, "book par"=w22:path, "IV path"=w38:path, "Field path"=w35:path)  [unwired: 4 in]
  n9 = flat-sequence {
    tunnel: w37 -> [w81]
    tunnel: [w81] -> w36
    frame #0 {
      n10 = Current VI's Path() -> (path=w82:path)
      n11 = local write "Current VI path"(w82) -> ()
    }
  }
  n12 = local read "Chan 1"() -> (w20:bool)
  n13 = local read "Chan 2"() -> (w19:bool)
  n14 = local read "Chan 3"() -> (w18:bool)
  n15 = Divide(x="Current Start uA", y="Current output Scale factor") -> (x/y=w54:dbl)
  n16 = Divide(x="Current Step uA", y="Current output Scale factor") -> (x/y=w53:dbl)
  n17 = Divide(x="Current Range uA", y="Current output Scale factor") -> (x/y=w52:dbl)
  n18 = Build Array(w20, w19, w18) -> (w17:bool[])
  n19 = Boolean To (0,1)(Boolean=w17) -> (0, 1=w16:i16[])
  n20 = Add Array Elements(numeric array=w16) -> (sum=w15:i16)
  n21 = call "Field sweep Generator.vi"("Ramp type"="Ramp type", "Ramp up first T"="Ramp up first T", "Field Radius"=w52, "Field step"=w53, "Field Origin"=w54) -> ("output array"=w26:dbl[])  [unwired: 6 in]
  n22 = call "Field sweep Generator.vi"("Ramp type"="Ramp type 2", "Ramp up first T"="Ramp up first T 2", "Field Radius"="Field Radius mT", "Field step"="Field step mT", "Field Origin"="Field Origin mT") -> ("output array"=w10:dbl[])  [unwired: 6 in]
  n23 = call "SaveControlValues.vi"("XML File Path"=w39, "error in (no error)"=w36) -> ("error out"=w34:errorcluster)  [unwired: 8 in]
  n24 = Multiply(x="Current output Scale factor", y=w26) -> (x*y=w8:dbl[])
  n25 = Increment(x=w15) -> (x+1=w14:i16)
  n26 = call-poly <vilib>:"Write Delimited Spreadsheet.vi"("file path (dialog if empty)"=w35, "format (%.3f)"=w28, "1D data"=w10, "error in (no error)"=w34) -> ("new file path (Not A Path if cancelled)"=w27:path, "error out"=w24:errorcluster)  [unwired: 10 in]
  n27 = Build Array(w14) -> (w13:i16[])
  n28 = To Double Precision Float(number=w13) -> (double precision float=w12:dbl[])
  n29 = call-poly <vilib>:"Write Delimited Spreadsheet.vi"("file path (dialog if empty)"=w27, "format (%.3f)"=w28, "1D data"=w8, "append to file? (new file:F)"=TRUE, "error in (no error)"=w24) -> ("error out"=w21:errorcluster)  [unwired: 9 in, 1 out]
  n30 = call-poly <vilib>:"Write Delimited Spreadsheet.vi"("file path (dialog if empty)"=w22, "format (%.3f)"="%d", "1D data"=w12, "error in (no error)"=w21) -> ("error out"=w11:errorcluster)  [unwired: 10 in, 1 out]
  n31 = call "Start cRIO DAQ.vi"("error in (no error)"=w11, "cRIO IP"="cRIO IP") -> ("error out"=w51:errorcluster, "vi reference"=w61:refnum<vi>, "application reference"=w62:refnum<vi>, "DAQ_AI_Reader endpoint"=w48:refnum<k21>, "DAQ_CMD_Writer endpoint"=w49:refnum<k21>)  [unwired: 5 in]
  n32 = for {
    tunnel: "AO Channel" -> [w110]
    tunnel: w26 -> [w109]
    tunnel: w49 -> [w108]
    tunnel: w48 -> [w107]
    tunnel: "Reading Average times" -> [w106]
    tunnel: w38 -> [w101]
    tunnel: w10 -> [w103] mode=indexing
    tunnel: w51 -> [w84]
    tunnel: [w96] -> w47
    tunnel: "Field Rate mT per sec" -> [w104]
    tunnel: "Magnet Device Select" -> [w86]
    i -> [w92]
    stop <- "stop" stop-if-true
    n33 = flat-sequence {
      tunnel: w84 -> [w112]
      tunnel: [w112] -> w83
      frame #0 {
        w111 = cluster{dbl[], dbl[]}[] []
        n34 = local write "I vs R"(w111) -> ()
        n35 = local write "I vs AI"(w111) -> ()
      }
    }
    n36 = Equal?(x=0, y=w92) -> (x = y?=w90:bool)
    n37 = Select(t=TRUE ("Init"), s=w90, f=FALSE) -> (s? t:f=w87:bool)
    n38 = call "set single axis Field Module.vi"("Field Device Select"=w86, "error in (no error)"=w83, "Init"=w87, "Field Target mT or dBm"=w103, "Exec"=TRUE, "Field Rate mT per sec"=w104, "final"=FALSE) -> ("error out"=w102:errorcluster)  [unwired: 12 in]
    n39 = for {
      tunnel: w102 -> [w155]
      tunnel: w108 -> [w154]
      tunnel: w110 -> [w153]
      tunnel: w109 -> [w147] mode=indexing
      tunnel: w107 -> [w151]
      tunnel: w106 -> [w146]
      tunnel: [w121] -> w95 mode=indexing
      i -> [w143]
      stop <- w139 stop-if-true
      n40 = call "cRIO Output voltage.vi"("Voltage"=w147, "AO Channel"=w153, "error in (no error)"=w155, "DAQ_CMD_Writer endpoint"=w154) -> ("error out"=w150:errorcluster, "DAQ_CMD_Writer endpoint out"=w152:refnum<k21>)  [unwired: 6 in]
      n41 = Equal?(x=0, y=w143) -> (x = y?=w142:bool)
      n42 = case shown="True" w142 {
        tunnel: "Delay Time s" -> [w174 _]
        tunnel: [w174 5.0 ("Delay Time s")] -> w140
        frame False {
        }
        frame True {
        }
      }
      n43 = local read "Current output Scale factor"() -> (w148:dbl)
      n44 = call "Time Delay"("error in (no error)"=w150, "Delay Time (s)"=w140) -> ("error out"=w149:errorcluster)  [unwired: 9 in]
      n45 = Multiply(x=w148, y=w147) -> (x*y=w119:dbl)
      n46 = call "cRIO Input voltage.vi"("DAQ_AI_Reader endpoint"=w151, "Average"=w146, "error in (no error)"=w149, "DAQ_CMD_Writer endpoint"=w152) -> ("error out"=w138:errorcluster, "output cluster"=w131:T2)  [unwired: 5 in, 1 out]
      n47 = call "cRIO AI data1.vi"("I"=w119, "Input cluster"=w131, "error in (no error)"=w138, "Chan 0"=TRUE, "Scale factor0"="Scale factor0", "Chan 1"="Chan 1", "Scale factor1"="Scale factor1", "Chan 2"="Chan 2", "Scale factor2"="Scale factor2", "Chan 3"="Chan 3", "Scale factor3"="Scale factor3") -> ("Output data"=w129:dbl[], "error out"=w125:errorcluster)  [unwired: 7 in]
      n48 = local read "Lockin 1"() -> (w127:bool)
      n49 = Array Subset(array=w129, index=1) -> (w126:dbl[])  [unwired: 1 in]
      n50 = case shown="True" w127 {
        tunnel: w125 -> [w166 w172]
        tunnel: [w166 w169] -> w124
        tunnel: w126 -> [w167 w171]
        tunnel: [w167 w170] -> w122
        tunnel: [0.0 ("R") w168] -> w118
        frame False {
        }
        frame True {
          n51 = local read "Lockin address 1"() -> (w173:string)
          n52 = call "Read XY.vi"("error in (no error)"=w172, "VISA resource name"=w173) -> ("error out"=w169:errorcluster, "R"=w168:dbl)  [unwired: 5 in, 3 out]
          n53 = Insert Into Array(array=w171, new element=w168) -> (w170:dbl[])  [unwired: 1 in]
        }
      }
      n54 = local read "I vs AI"() -> (w130:cluster{"Y":dbl[], "Y":dbl[]}[])
      n55 = call "add data to plot 1.vi"("Input graph"=w130, "Input Y array"=w126, "x"=w119) -> ("Output graph"=→"I vs AI":cluster{dbl[], dbl[]}[])  [unwired: 7 in, 1 out]
      n56 = local read "Lockin 2"() -> (w123:bool)
      n57 = case shown="True" w123 {
        tunnel: w124 -> [w157 w163]
        tunnel: [w157 w160] -> _
        tunnel: w122 -> [w158 w162]
        tunnel: [w158 w161] -> w121
        tunnel: [0.0 ("R") w159] -> w117
        frame False {
        }
        frame True {
          n58 = local read "Lockin address 2"() -> (w164:string)
          n59 = call "Read XY.vi"("error in (no error)"=w163, "VISA resource name"=w164) -> ("error out"=w160:errorcluster, "R"=w159:dbl)  [unwired: 5 in, 3 out]
          n60 = Insert Into Array(array=w162, new element=w159) -> (w161:dbl[])  [unwired: 1 in]
        }
      }
      n61 = Build Array(w118, w117) -> (w116:dbl[])
      n62 = local read "I vs R"() -> (w120:cluster{"Y":dbl[], "Y":dbl[]}[])
      n63 = call "add data to plot 1.vi"("Input graph"=w120, "Input Y array"=w116, "x"=w119) -> ("Output graph"=→"I vs R":cluster{dbl[], dbl[]}[])  [unwired: 7 in, 1 out]
      n64 = local read "stop"() -> (w139:bool)
    }
    n65 = Transpose 2D Array(2D array=w95) -> (transposed array=w85:dbl[][])
    n66 = call-poly <vilib>:"Write Delimited Spreadsheet.vi"("file path (dialog if empty)"=w101, "format (%.3f)"="%.9e", "2D data"=w85, "append to file? (new file:F)"=TRUE, "transpose? (no:F)"=FALSE, "delimiter (\\t)"="\t" ("delimiter (\\t)")) -> ("error out"=w96:errorcluster)  [unwired: 8 in, 1 out]
    "Current Field mT" <- w103
  }
  n67 = call "Stop cRIO DAQ.vi"("DAQ_AI_Reader endpoint"=w48, "DAQ_CMD_Writer endpoint"=w49, "error in (no error)"=w47, "VI reference"=w61, "application reference"=w62) -> ("error out"=→"error out":errorcluster)  [unwired: 6 in]
  "Name 0" <- "Channel name 0"
  "Name 1" <- "Channel name 1"
  "Name 2" <- "Channel name 2"
  "Name 3" <- "Channel name 3"
